vi "decimate data example.vi"() -> ()   [LabVIEW 2014]
uses:
  <vilib>/measure/NI_MABase.lvlib
panel:
  out "Y":dbl[](array[numeric])
  out "Waveform Chart 2":waveform(dbl)(graph)
  out "Waveform Chart":waveform(dbl)(graph)
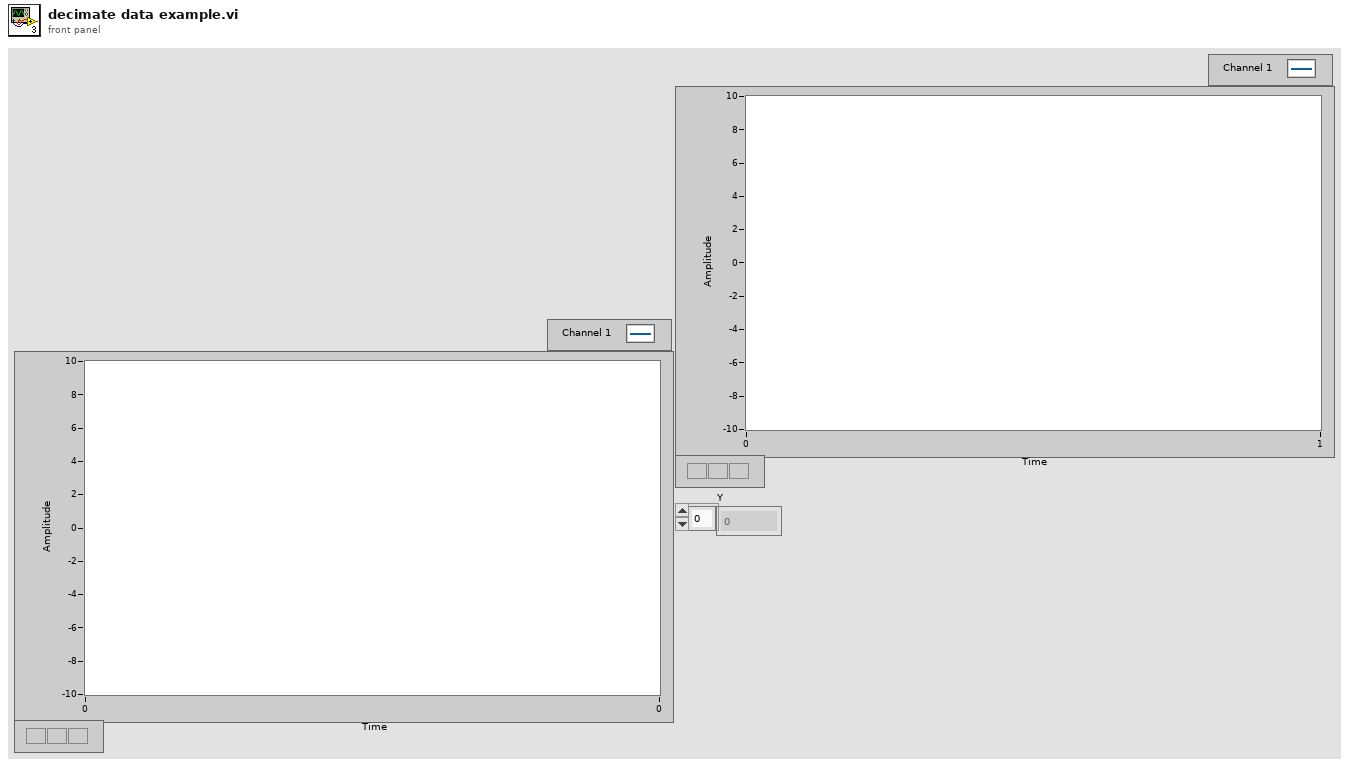
[diagram p1: front panel]
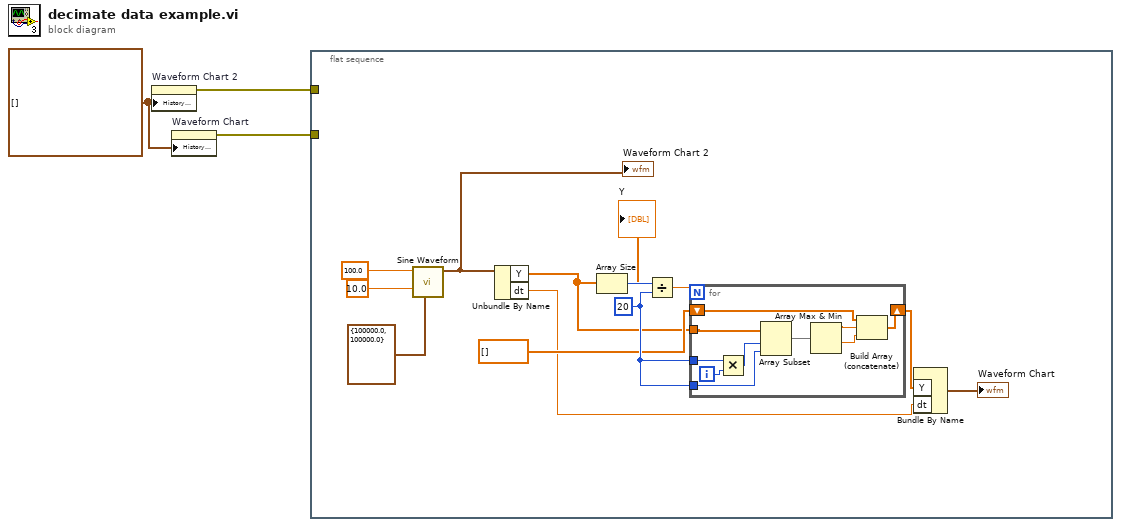
[diagram p0: block diagram]
diagram:
  w3 = waveform(dbl)[] [] ("History Data")
  n1 = property on="Waveform Chart 2" class="WFChart (strict)"("History Data"=w3) -> (error out=w2:errorcluster)  [unwired: 2 in, 1 out]
  n2 = property on="Waveform Chart" class="WFChart (strict)"("History Data"=w3) -> (error out=w1:errorcluster)  [unwired: 2 in, 1 out]
  n3 = flat-sequence {
    tunnel: w2 -> [_]
    tunnel: w1 -> [_]
    frame #0 {
      w12 = 20 ("y")
      n4 = call <vilib>:"Sine Waveform.vi"("sampling info"=cluster{"Fs":dbl, "#s":dbl} {"Fs"=100000.0, "#s"=100000.0}, "amplitude"=10.0, "frequency"=100.0) -> ("signal out"=w6:waveform(dbl))  [unwired: 7 in, 1 out]
      "Waveform Chart 2" <- w6
      n5 = Unbundle By Name(w6) -> ("Y"=w5:dbl[], "dt"=w4:dbl)
      "Y" <- w5
      n6 = Array Size(array=w5) -> (size(s)=w14:i32)
      n7 = Divide(x=w14, y=w12) -> (x/y=w13:dbl)
      n8 = for {
        N: w13 -> [_]
        tunnel: w5 -> [w25]
        tunnel: w12 -> [w23]
        tunnel: w12 -> [w21]
        shift-right: [w16] -> w10
        shift-left: dbl[] [] -> [w17]
        i -> [w24]
        n9 = Multiply(x=w23, y=w24) -> (x*y=w22:i32)
        n10 = Array Subset(array=w25, index=w22, length=w21) -> (w20:dbl[])
        n11 = Array Max & Min(array=w20) -> (max value=w18:dbl, min value=w19:dbl)  [unwired: 2 out]
        n12 = Build Array (concatenate)(w17, w18, w19) -> (w16:dbl[])
      }
      n13 = Bundle By Name("Y"=w10, "dt"=w4) -> (→"Waveform Chart":waveform(dbl))  [unwired: 1 in]
    }
  }
